vi "Read Base Description.vi"(11 "Mocha in":refnum<class "Whip.lvclass">) -> (2 "Description":string)   [LabVIEW 2013, in "Whip.lvclass"]
uses:
  Whip.lvclass
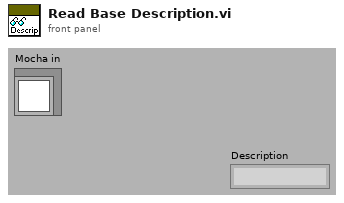
[diagram p1: front panel]
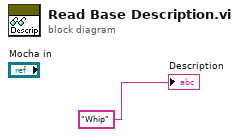
[diagram p0: block diagram]
diagram:
  "Description" <- "Whip" ("string")
